vi "Test3v4.vi"() -> ()   [LabVIEW 2013]
panel:
  out "appended array":string[][](array[string])
  out "index":i32
  out "*(type *) &x":string
  out "size(s)":i32
  out "hex integer string":string[](array[string])
  in  "error in":errorcluster
  out "error out":errorcluster
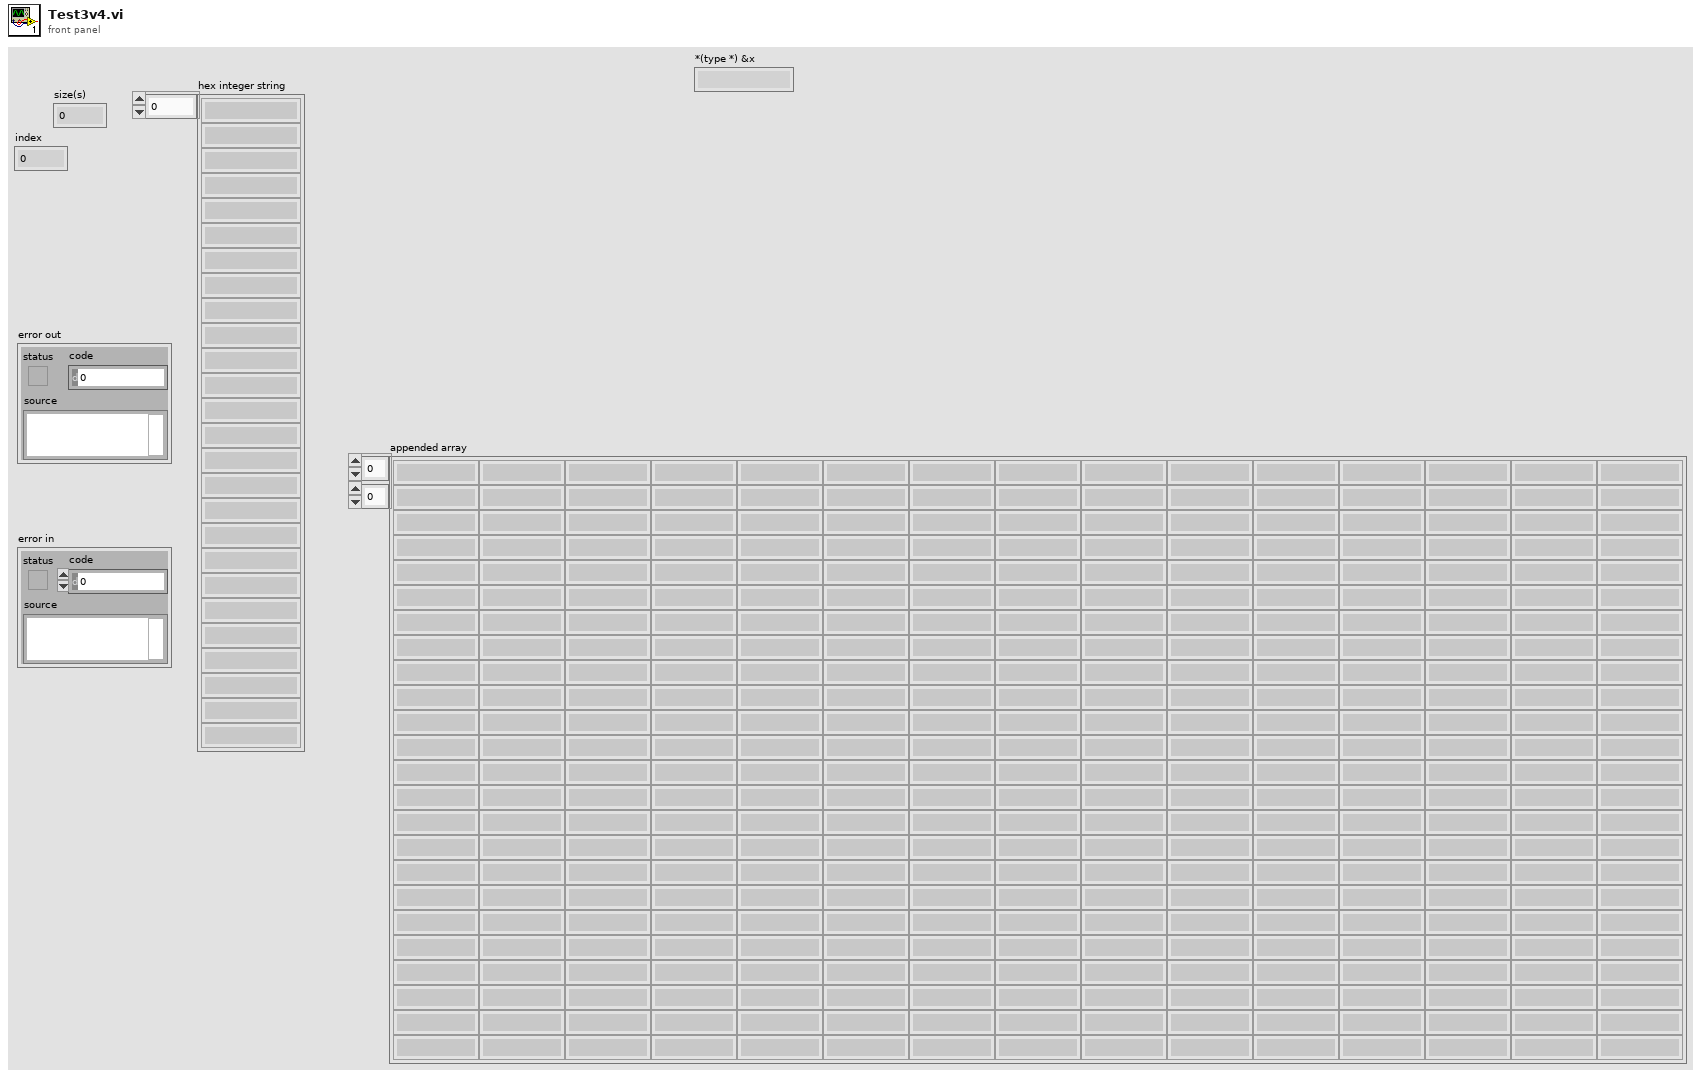
[diagram p1: front panel]
types:
  T1 = enum16{"big-endian, network order", "native, host order", "little-endian"}
  T2 = enum16{"open", "replace", "create", "open or create", "replace or create", "replace or create with confirmation"}
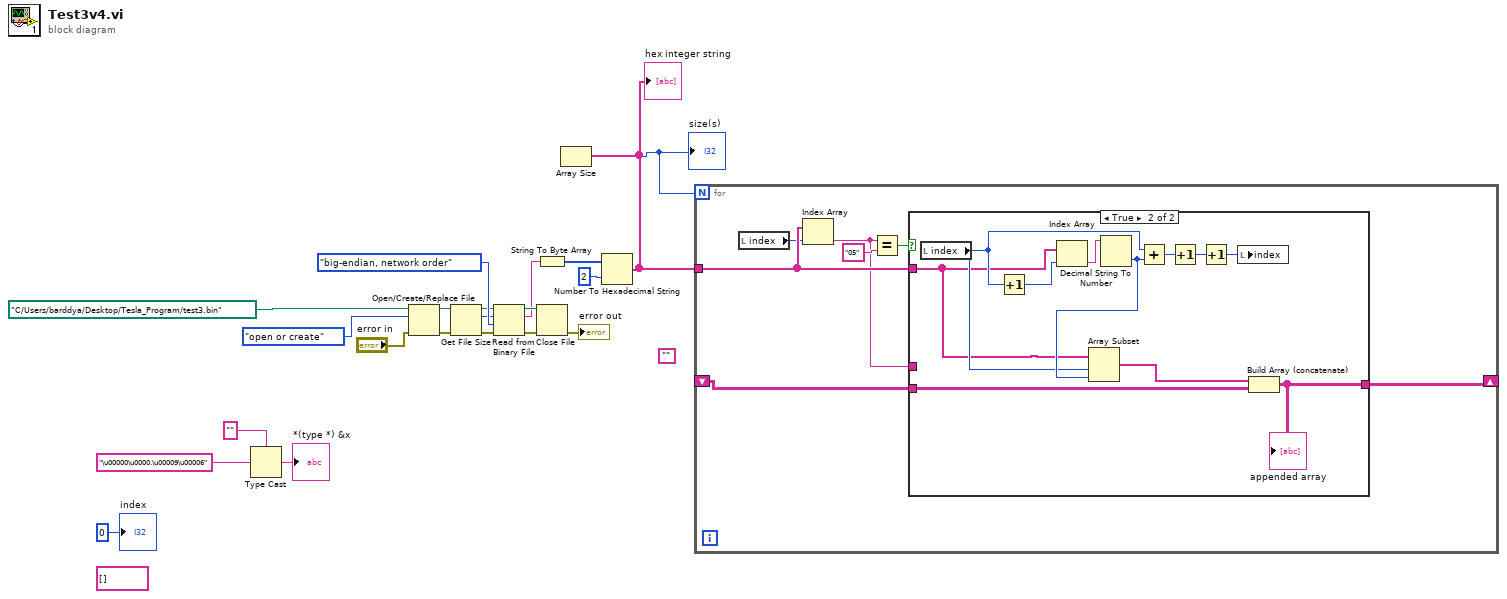
[diagram p0: block diagram]
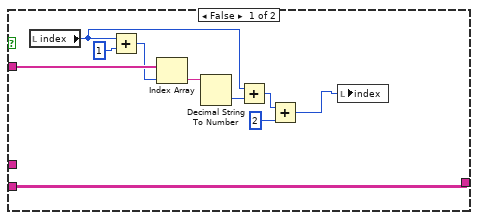
[diagram p2: hidden frame]
diagram:
  (unwired) ""
  (unwired) string[] [] ("subarray")
  n1 = Type Cast(type="", x="\u00000\u0000.\u00009\u00006") -> (*(type *) &x=→"*(type *) &x":string)
  n2 = Open/Create/Replace File(file path (use dialog)=path "C:/Users/barddya/Desktop/Tesla_Program/test3.bin", error in="error in", operation (0:open)=T2."open or create") -> (refnum out=w14:refnum<file>, error out=w12:errorcluster)  [unwired: 3 in, 1 out]
  n3 = Get File Size(file=w14, error in=w12) -> (refnum out=w13:refnum<file>, size (in bytes)=w10:i64, 0:w11:errorcluster)
  n4 = Read from Binary File(8:w11, 9:T1."big-endian, network order" ("byte order (0:big-endian, network order)"), 10:w10, 11:w13) -> (0:w17:errorcluster, 2:w9:string, 3:w15:refnum<file>)  [unwired: 2 in, 1 out]
  n5 = String To Byte Array(string=w9) -> (unsigned byte array=w8:u8[])
  n6 = Close File(refnum=w15, error in=w17) -> (error out=→"error out":errorcluster)  [unwired: 1 out]
  n7 = Number To Hexadecimal String(1:2, 2:w8) -> (0:w3:string[])
  "hex integer string" <- w3
  n8 = Array Size(array=w3) -> (size(s)=w1:i32)
  "size(s)" <- w1
  n9 = for {
    N: w1 -> [_]
    tunnel: w3 -> [w26]
    shift-right: [w23] -> _
    shift-left: _ -> [w22]
    n10 = local read "index"() -> (w24:i32)
    n11 = Index Array(array=w26, index=w24) -> (element=w25:string)
    n12 = Equal?(x=w25, y="05") -> (x = y?=w27:bool)
    n13 = case shown="True" w27 {
      tunnel: w26 -> [w36 w40]
      tunnel: w25 -> [_ _]
      tunnel: [w29 w39] -> w23
      tunnel: w22 -> [w29 w44]
      frame False {
        n14 = local read "index"() -> (w33:i32)
        n15 = Add(x=w33, y=1) -> (x+y=w34:i32)
        n16 = Index Array(array=w36, index=w34) -> (element=w38:string)
        n17 = Decimal String To Number(string=w38) -> (number=w37:i32)  [unwired: 2 in, 1 out]
        n18 = Add(x=w33, y=w37) -> (x+y=w32:i32)
        n19 = Add(x=w32, y=2) -> (x+y=w30:i32)
        n20 = local write "index"(w30) -> ()
      }
      frame True {
        n21 = local read "index"() -> (w41:i32)
        n22 = Increment(x=w41) -> (x+1=w46:i32)
        n23 = Index Array(array=w40, index=w46) -> (element=w47:string)
        n24 = Decimal String To Number(string=w47) -> (number=w42:i32)  [unwired: 2 in, 1 out]
        n25 = Array Subset(array=w40, index=w41, length=w42) -> (w45:string[])
        n26 = Add(x=w41, y=w42) -> (x+y=w48:i32)
        n27 = Increment(x=w48) -> (x+1=w49:i32)
        n28 = Increment(x=w49) -> (x+1=w43:i32)
        n29 = local write "index"(w43) -> ()
        n30 = Build Array (concatenate)(w45, w44) -> (w39:string[][])
        "appended array" <- w39
      }
    }
  }
  "index" <- 0
